vi "Monitor Data - All Runtime.vi"(8 "error in (no error)":errorcluster, 9 "Check Period (ms)":u32, 11 "RT - Analysis Data in":T1={"Accel Sensistivity"=[0.0, 0.0, 0.0], "Cutoff Frequncies"=[{"LP Passband"=0.0, "HP Stopband"=0.0, "LP Stopband"=0.0, "HP Passband"=0.0}, {"LP Passband"=0.0, "HP Stopband"=0.0, "LP Stopband"=0.0, "HP Passband"=0.0}, {"LP Passband"=0.0, "HP Stopband"=0.0, "LP Stopband"=0.0, "HP Passband"=0.0}], "APU Setup File"={"Sensor Info"=[], "Calibration Info"=[], "CMM Table 106"=[], "CMM Table 106B "=[], "Accel Config"=[], "Report Sheet 1"=[], "Report Sheet 2"=[], "Report Sheet 3"=[]}, "RepairLevel"=""} {"Cutoff Frequncies"."HP Passband" min=1.0 step=1.0 format="%#.4f"; "Cutoff Frequncies"."LP Stopband" min=1.0 step=1.0 format="%#.4f"; "Cutoff Frequncies"."HP Stopband" min=1.0 step=1.0 format="%#.4f"; "Cutoff Frequncies"."LP Passband" min=1.0 step=1.0 format="%#.4f"}) -> (0 "error out":errorcluster)   [LabVIEW 2018, in "RT - Analysis.lvlib"]
uses:
  RT - Analysis.lvlib
  Private Controls/RT-Analysis Data.ctl
  Modules/Testing UI 3/Private Controls/Cutoff Frequency.ctl
  Modules/Testing UI 3/Testing UI 3.lvlib
  Top Level/Shared Controls/APU Setup File.ctl
panel:
  # "Highpass Cutoff Frequency"
  # "Lowpass Cutoff Frequency"
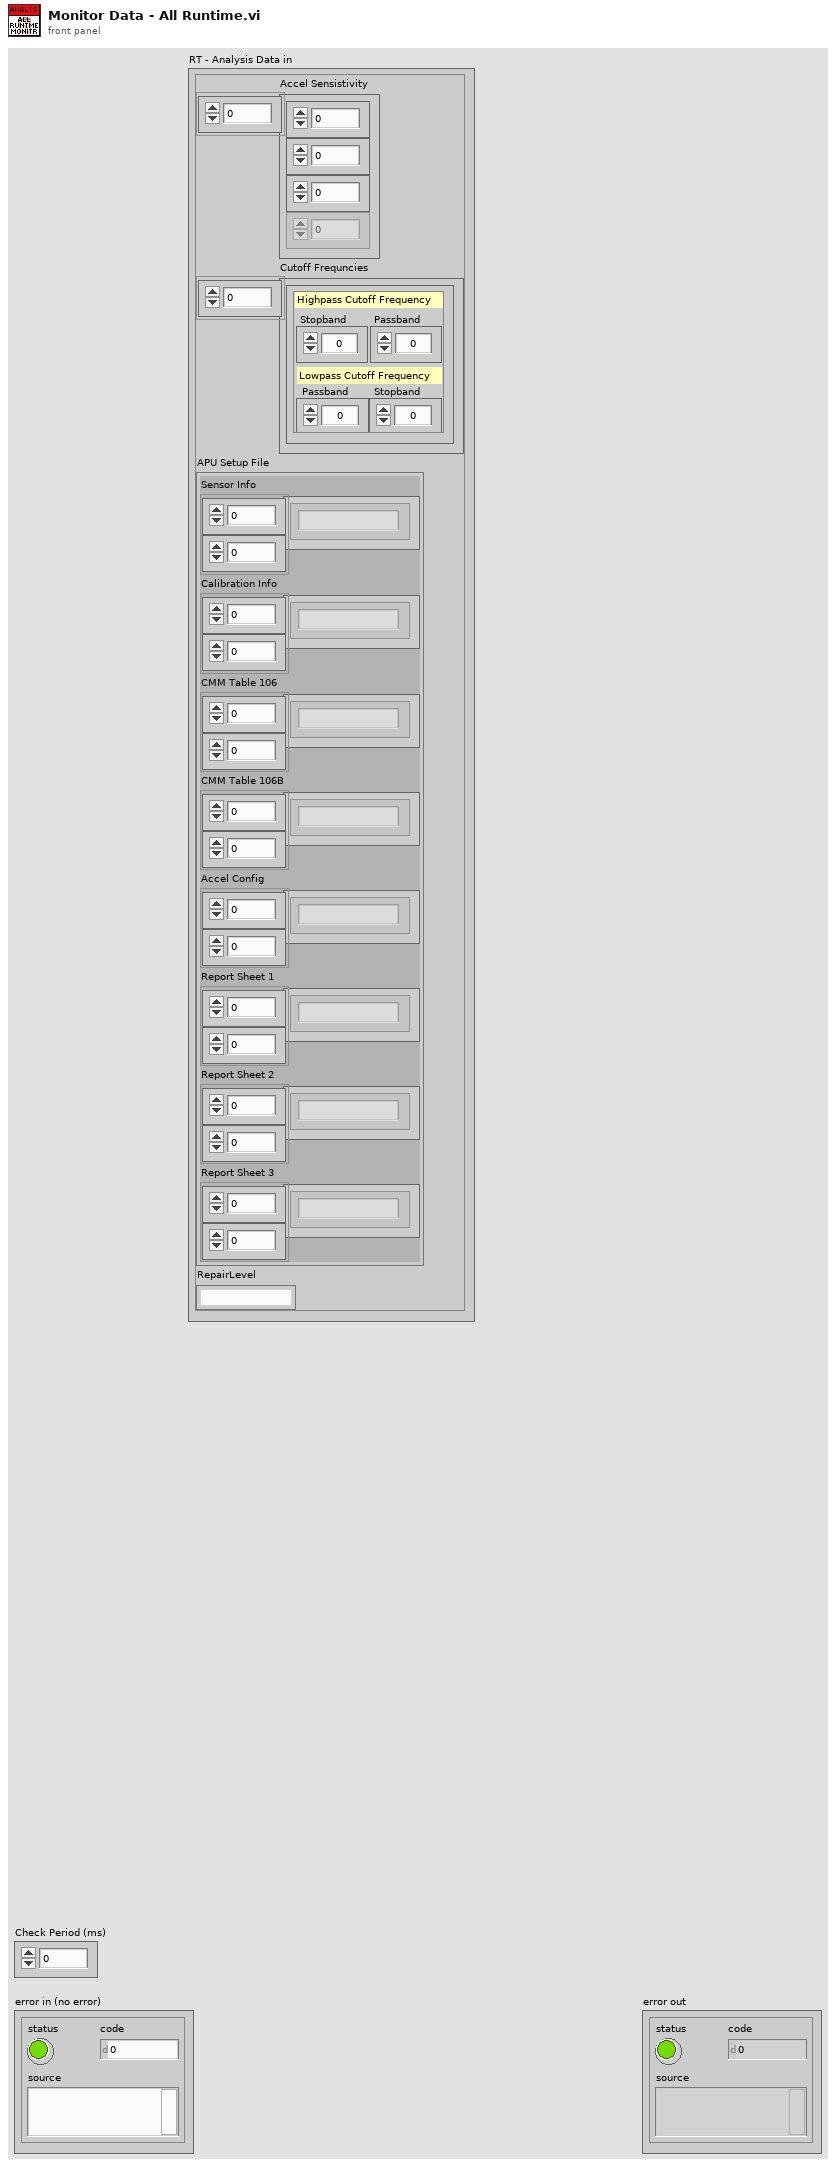
[diagram p1: front panel]
types:
  T1 = typedef "RT - Analysis.lvlib/RT-Analysis Data.ctl" = cluster{"Accel Sensistivity":dbl[], "Cutoff Frequncies":T2[], "APU Setup File":T3, "RepairLevel":string}
  T2 = typedef "Testing UI 3.lvlib/Cutoff Frequency.ctl" = cluster{"LP Passband":dbl, "HP Stopband":dbl, "LP Stopband":dbl, "HP Passband":dbl}
  T3 = typedef "APU Setup File.ctl" = cluster{"Sensor Info":string[][], "Calibration Info":string[][], "CMM Table 106":string[][], "CMM Table 106B ":string[][], "Accel Config":string[][], "Report Sheet 1":string[][], "Report Sheet 2":string[][], "Report Sheet 3":string[][]}
  T4 = typedef "Post-Analysis Data.ctl" = cluster{"Calibrated Data":cluster{"00-00-9205 Calib":dbl[], "00-01-9205 Calib":dbl[], "01-00-9213 Calib":dbl[], "01-01-9213 Calib":dbl[], "01-02-9213 Calib":dbl[], "02-02-9219 Calib":dbl[], "02-03-9227 Calib":dbl[], "00-02-9234 Calib":dbl[], "00-03-9402 Calib":dbl[], "02-05-9205 Calib":dbl[], "02-04-9871 2DArray":dbl[][]}, "Calculated Data":T5, "Indicator Data":cluster{"00-02-9234 Peak Vel (in/sec)":dbl[]}}
  T5 = typedef "Calculated Data.ctl" = cluster{"C.00":dbl, "C.01":dbl, "C.02":dbl, "C.03":dbl, "C.04":dbl, "C.05":dbl, "C.06":dbl, "C.07":dbl, "C.08":dbl, "C.09":dbl, "C.10":dbl, "C.11":dbl, "C.12":dbl, "C.13":dbl, "C.14":dbl, "C.15":dbl, "C.16":dbl, "C.17":dbl, "C.18":dbl, "C.19":dbl, "C.20":dbl, "C.21":dbl, "C.22":dbl, "C.23":dbl, "C.24":dbl, "C.25":dbl, "C.26":dbl, "C.27":dbl, "C.28":dbl, "C.29":dbl, "C.30":dbl, "C.31":dbl, "C.32":dbl, "C.33":dbl, "C.34":dbl, "C.35":dbl, "C.36":dbl, "C.37":dbl, "C.38":dbl, "C.39":dbl, "C.40":dbl, "C.41":dbl, "C.42":dbl, "C.43":dbl, "C.44":dbl, "C.45":dbl, "C.46":dbl, "C.47":dbl, "C.48":dbl, "C.49":dbl, "C.50":dbl, "C.51":dbl, "C.52":dbl, "C.53":dbl, "C.54":dbl, "C.56":dbl}
  T6 = typedef "RT - Analysis.lvlib/Parsed Data Arrays.ctl" = cluster{"[Parsed Tags]":T7[], "[VData out]":variant[], "[Whole Tags]":string[]}
  T7 = typedef "Parsed Tag Cluster.ctl" = cluster{"Whole Tag":string, "# of Sections":u8, "Chassis":u8, "Slot":u8, "Module":string, "Channel":u8, "SubChannel":u8}
  T8 = cluster{"Post-Analysis Data":T4, "Parsed Data Arrays":T6}
  T9 = typedef "RT - Analysis.lvlib/Alert Data.ctl" = cluster{"Tag":string, "Value":dbl, "Alerts":bool[], "Thresh Val":dbl, "Thresh Len":dbl, "Thresh Type":enum16{"Neither", "Max", "Min"}}
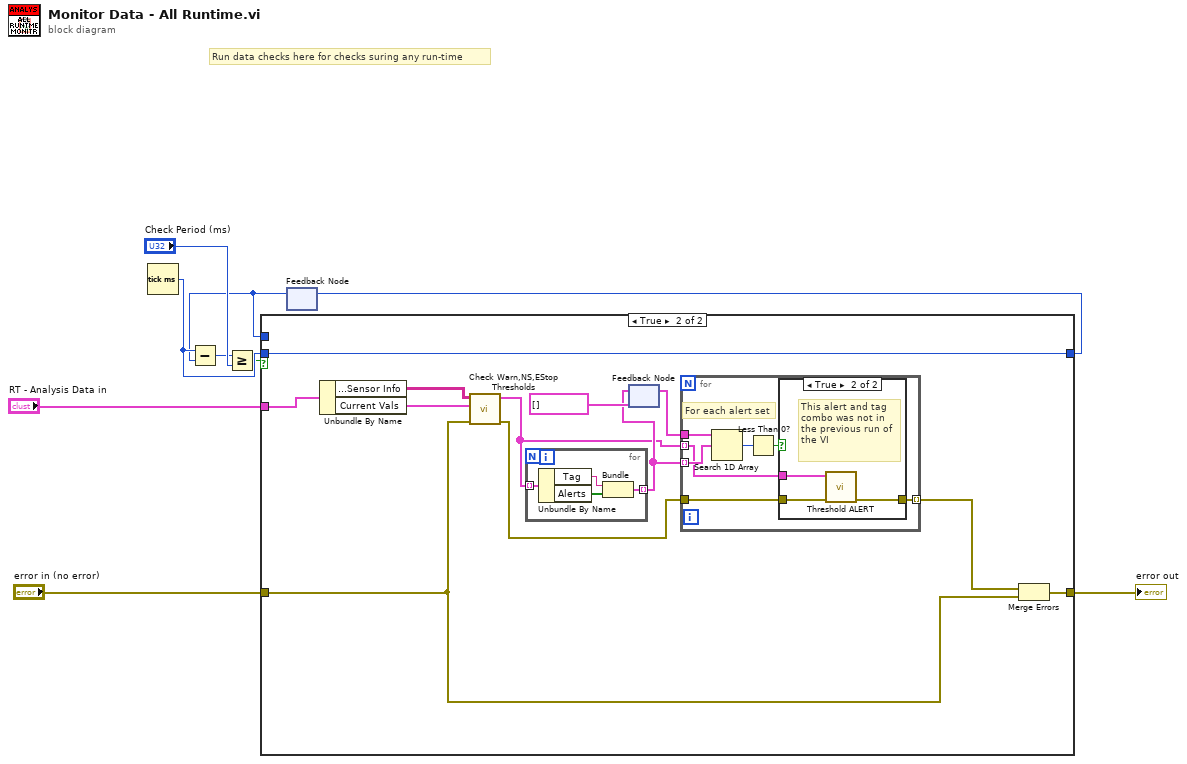
[diagram p0: block diagram]
diagram:
  # "Run data checks here for checks suring any run-time"
  n1 = Tick Count (ms)() -> (millisecond timer value=w9:u32)
  n2 = feedback #1() -> (w6:u32)  [unwired: 1 in]
  n3 = Subtract(x=w9, y=w6) -> (x-y=w5:u32)
  n4 = Greater Or Equal?(x=w5, y="Check Period (ms)") -> (x >= y?=w7:bool)
  n5 = case shown="True" w7 {
    tunnel: "error in (no error)" -> [w10 w13]
    tunnel: [w10 w18] -> w3
    tunnel: [w11 w23] -> w4
    tunnel: w6 -> [w11 _]
    tunnel: w9 -> [_ w23]
    tunnel: "RT - Analysis Data in" -> [_ w12]
    frame False {
    }
    frame True {
      n6 = Unbundle By Name(w12) -> ("APU Setup File.Sensor Info"=w15:string[][], "Current Vals"=w14:T8)
      n7 = call "Check Warn,NS,EStop Thresholds.vi"("error in (no error)"=w13, "Current Vals"=w14, "[[APU Sensor Info]]"=w15) -> ("error out"=w19:errorcluster, "[Tags and Alerts]"=w16:T9[])  [unwired: 7 in]
      n8 = for {
        tunnel: w16 -> [w27] mode=indexing
        tunnel: [w25] -> w17 mode=indexing
        n9 = Unbundle By Name(w27) -> ("Tag"=w24:string, "Alerts"=w26:bool[])
        n10 = Bundle("Tag"=w24, "Alerts"=w26) -> (w25:cluster{"Tag":string, "Alerts":bool[]})  [unwired: 1 in]
      }
      n11 = feedback #2(cluster{"Tag":string, "Alerts":bool[]}[] []) -> (w21:cluster{"Tag":string, "Alerts":bool[]}[])
      n12 = feedback-in #2(w17) -> ()
      n13 = for {
        tunnel: [w30] -> w22 mode=indexing
        tunnel: w19 -> [w31]
        tunnel: w16 -> [w28] mode=indexing
        tunnel: w21 -> [w34]
        tunnel: w17 -> [w29] mode=indexing
        # "For each alert set"
        n14 = Search 1D Array(1D array=w34, element=w29) -> (index of element=w33:i32)  [unwired: 1 in]
        n15 = Less Than 0?(x=w33) -> (x < 0?=w32:bool)
        n16 = case shown="True" w32 {
          tunnel: w28 -> [_ w36]
          tunnel: w31 -> [w35 w38]
          tunnel: [w35 w37] -> w30
          frame False {
          }
          frame True {
            # "This alert and tag combo was not in the previous run of the VI"
            n17 = call "Threshold ALERT.vi"("error in (no error)"=w38, "Alert Data"=w36) -> ("error out"=w37:errorcluster)  [unwired: 9 in]
          }
        }
      }
      n18 = Merge Errors(w22, w13) -> (w18:errorcluster)
    }
  }
  "error out" <- w3
  n19 = feedback-in #1(w4) -> ()
